vi "Read ISO Format.vi"(11 "DateTime.ISO8601 in":refnum<class "DateTime.ISO8601.lvclass">) -> (2 "ISO Format":T1, 3 "DateTime.ISO8601 out":refnum<class "DateTime.ISO8601.lvclass">)   [LabVIEW 2013, in "DateTime.ISO8601.lvclass"]
uses:
  DateTime.ISO8601.lvclass
  ISO8601 Date Formats.ctl
  DateTime.ISO8601.lvclass/DateTime.ISO8601.ctl
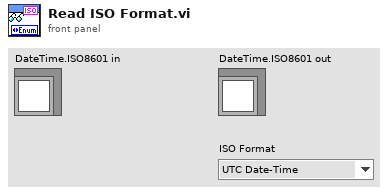
[diagram p1: front panel]
types:
  T1 = typedef "ISO8601 Date Formats.ctl" = enum16{"UTC Date-Time", "ISO Time", "Date", "Calendar Month", "Week", "Week-Day", "Month-Day", "Ordinal Date"}
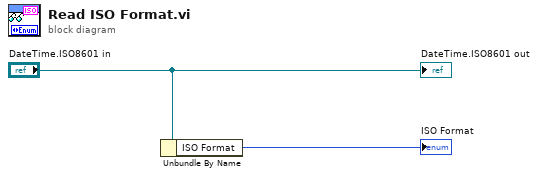
[diagram p0: block diagram]
diagram:
  n1 = Unbundle By Name("DateTime.ISO8601 in") -> ("ISO Format"=→"ISO Format":T1)
  "DateTime.ISO8601 out" <- "DateTime.ISO8601 in"
